vi "完全平方数(for新增功能）.vi"(11 "范围":i32=100) -> (3 "平方数":i32[](array[numeric]))   [LabVIEW 2012]
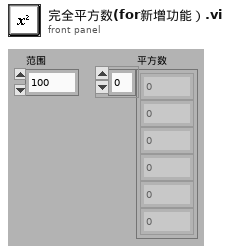
[diagram p1: front panel]
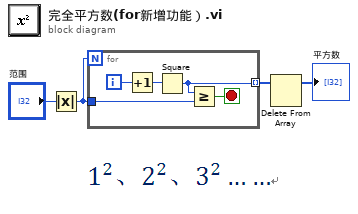
[diagram p0: block diagram]
diagram:
  n1 = Absolute Value(x="范围") -> (abs(x)=w1:i32)
  n2 = for {
    N: w1 -> [_]
    tunnel: w1 -> [w9]
    tunnel: [w6] -> w4 mode=indexing
    i -> [w8]
    stop <- w5 stop-if-true
    n3 = Increment(x=w8) -> (x+1=w7:i32)
    n4 = Square(x=w7) -> (x^2=w6:i32)
    n5 = Greater Or Equal?(x=w6, y=w9) -> (x >= y?=w5:bool)
  }
  n6 = Delete From Array(array=w4) -> (array with subset deleted=→"平方数":i32[])  [unwired: 2 in, 1 out]
